vi "Read Valve Output.vi"(8 "error in (no error)":errorcluster, 10 "Node (3)":u8=3 caption="Node" min=3 max=128 step=1, 11 "VISA resource name":refnum<visa-resource-name>) -> (0 "error out":errorcluster, 1 "Valve Output A":dbl format="%.3f", 2 "Valve Output Percentage":dbl format="%#.2g", 3 "VISA resource name out":refnum<visa-resource-name>)   [LabVIEW 2024, in "Bronkhorst FLOW-BUS.lvlib"]
doc: "Reads the controller output going to the DAC for driving the valve. \nRange: 0...16777215 ( 0...300mA)."
uses:
  Bronkhorst FLOW-BUS.lvlib
  Private/FLOW-BUS RW.ctl
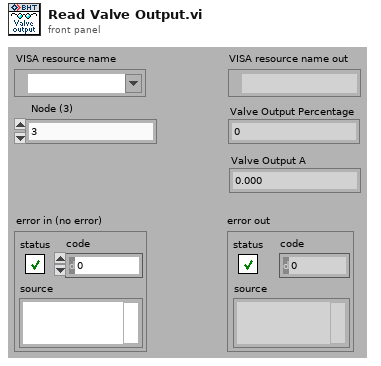
[diagram p1: front panel]
types:
  T1 = typedef "Bronkhorst FLOW-BUS.lvlib/FLOW-BUS RW.ctl" = cluster{"Node Address (3)":u8, "Communication Command":enum16{"Status message", "Send parameter with destination address and 00 response", "Send parameter with destination address", "Request parameter"}, "Process (0)":u16, "Parameter (0)":u16, "Data Type (0: Character)":enum16{"Character", "Integer", "Float or Long", "String"}, "Data for Char or Int (0)":u32, "Data for Float or Long (0)":sgl, "Data for String":string, "Length of Requested String (0)":u8}
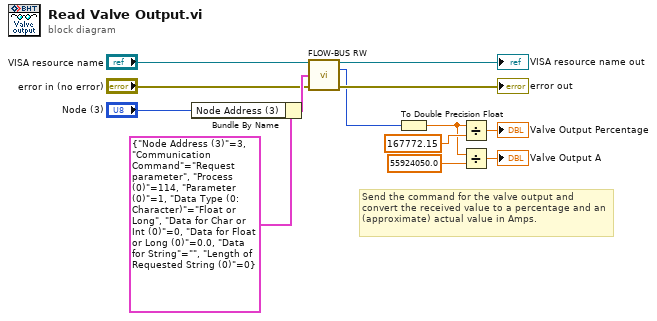
[diagram p0: block diagram]
diagram:
  # "Send the command for the valve output and convert the received value to a percentage and an (approximate) actual value in Amps."
  n1 = Bundle By Name(cluster=T1 {"Node Address (3)"=3, "Communication Command"=enum."Request parameter", "Process (0)"=114, "Parameter (0)"=1, "Data Type (0: Character)"=enum."Float or Long", "Data for Char or Int (0)"=0, "Data for Float or Long (0)"=0.0, "Data for String"="", "Length of Requested String (0)"=0} ("FLOW-BUS Command Settings"), "Node Address (3)"="Node (3)") -> (w8:T1)
  n2 = call "FLOW-BUS RW.vi"("VISA resource name"="VISA resource name", "FLOW-BUS Command Settings"=w8, "error in (no error)"="error in (no error)") -> ("VISA resource name out"=→"VISA resource name out":refnum<visa-resource-name>, "Requested Char, Int or Long"=w2:u32, "error out"=→"error out":errorcluster)  [unwired: 8 in, 2 out]
  n3 = To Double Precision Float(number=w2) -> (double precision float=w9:dbl)
  n4 = Divide(x=w9, y=167772.15) -> (x/y=→"Valve Output Percentage":dbl)
  n5 = Divide(x=w9, y=55924050.0) -> (x/y=→"Valve Output A":dbl)
